vi "Grab Cal Inst Waveforms.vi"(11 "all rows":string[][](array[string])) -> (1 "Current Waverform":waveform(dbl)(graph), 2 "Voltage Waveform":waveform(dbl)(graph), 3 "Resulting Time Stamp":timestamp)   [LabVIEW 2013]
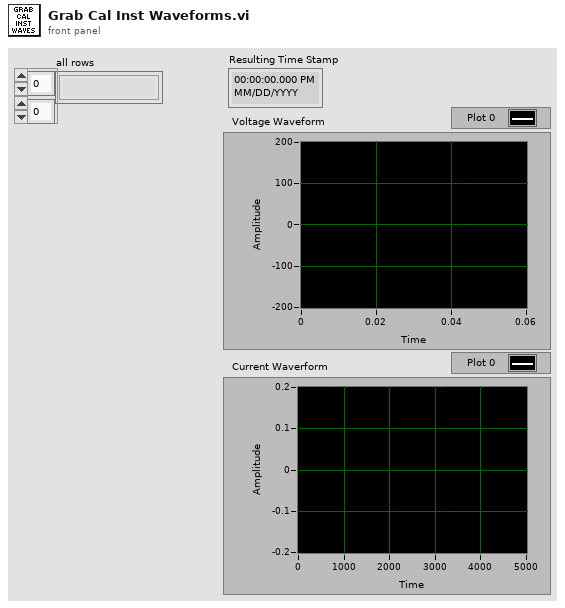
[diagram p1: front panel]
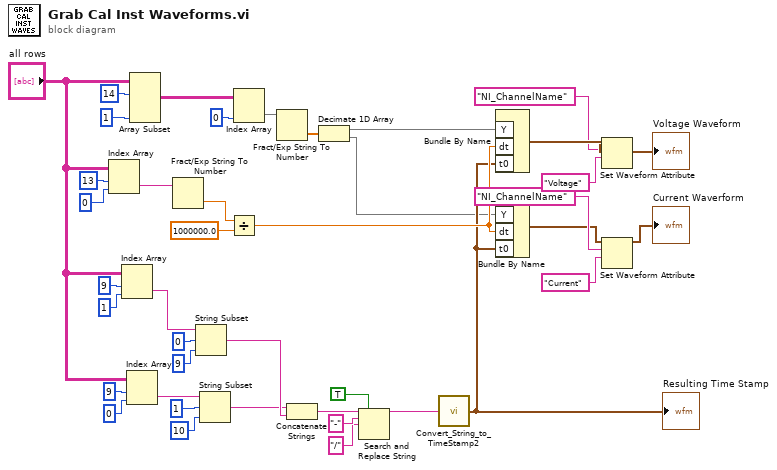
[diagram p0: block diagram]
diagram:
  n1 = Index Array(array="all rows", index (row)=13 ("disabled index (row)"), index (col)=0 ("disabled index (col)")) -> (element=w39:string)
  n2 = Index Array(array="all rows", index (row)=9, index (col)=1 ("disabled index (col)")) -> (element=w23:string)
  n3 = Index Array(array="all rows", index (row)=9, index (col)=0 ("disabled index (col)")) -> (element=w26:string)
  n4 = Array Subset(array="all rows", index (row)=14 ("index"), length (col)=1 ("length")) -> (w33:string[][])  [unwired: 2 in]
  n5 = Fract/Exp String To Number(string=w39) -> (number=w40:dbl)  [unwired: 3 in, 1 out]
  n6 = String Subset(string=w23, offset (0)=0, length (rest)=9 ("length (rest)")) -> (substring=w22:string)
  n7 = String Subset(string=w26, offset (0)=1, length (rest)=10 ("length (rest)")) -> (substring=w21:string)
  n8 = Divide(x=w40, y=1000000.0) -> (x/y=w12:dbl)
  n9 = Index Array(array=w33, index (col)=0 ("disabled index (col)")) -> (element=w35:string[])  [unwired: 1 in]
  n10 = Fract/Exp String To Number(string=w35) -> (number=w36:dbl[])  [unwired: 3 in, 1 out]
  n11 = Concatenate Strings(w21, w22) -> (w18:string)
  n12 = Decimate 1D Array(w36) -> (w10:dbl[], w9:dbl[])
  n13 = Search and Replace String(replace all?=TRUE ("replace all? (F)"), input string=w18, search string="-", replace string="/" ("replace string (\"\")")) -> (result string=w14:string)  [unwired: 4 in, 3 out]
  n14 = call "Convert_String_to_TimeStamp2.vi"("date/time string"=w14) -> ("Resulting Time Stamp"=w11:timestamp)
  "Resulting Time Stamp" <- w11
  n15 = Bundle By Name("Y"=w10, "dt"=w12, "t0"=w11) -> (w8:waveform(dbl))  [unwired: 1 in]
  n16 = Bundle By Name("Y"=w9, "dt"=w12, "t0"=w11) -> (w1:waveform(dbl))  [unwired: 1 in]
  n17 = Set Waveform Attribute(5:"Voltage" ("name"), 6:"NI_ChannelName" ("name"), 7:w8) -> (3:→"Voltage Waveform":waveform(dbl))  [unwired: 1 in, 2 out]
  n18 = Set Waveform Attribute(5:"Current" ("name"), 6:"NI_ChannelName" ("name"), 7:w1) -> (3:→"Current Waverform":waveform(dbl))  [unwired: 1 in, 2 out]
